vi "Test Process Register For Broadcast Throws Error if Process Uninitialized.vi"(8 "error in (no error)":errorcluster, 11 "Process Test in":refnum<class "Process Dev Test.lvclass">) -> (0 "error out":errorcluster, 3 "Process Test out":refnum<class "Process Dev Test.lvclass">)   [LabVIEW 2020, in "Process Dev Test.lvclass"]
uses:
  Process Dev Test.lvclass
  C:/Program Files (x86)/National Instruments/LabVIEW 2020/vi.lib/Astemes/LUnit/Test Case.lvclass
  source/Framework/Process/Process.lvclass
  source/Framework/Process/Process.lvclass/Process.ctl
  <vilib>/Astemes/LUnit/Test Case.lvclass/Test Case.ctl
  <vilib>/Astemes/LUnit/LUnit Assertion Result.lvclass/LUnit Assertion Result.ctl
  <vilib>/Astemes/LUnit/LUnit Test Case Result.lvclass/LUnit Test Case Result.ctl
  <vilib>/Astemes/LUnit/LUnit Method Result.lvclass/LUnit Method Result.ctl
  source/Framework/Process/Public/Lifecycle/Get Lifecycle State.vi
  <vilib>/Astemes/LUnit/Palette/Fail.vi
  <vilib>/Astemes/LUnit/Palette/Pass.vi
  <vilib>/Astemes/LUnit/Set Assertion Type.vi
  <vilib>/Utility/error.llb/Clear Errors.vi
  <vilib>/Astemes/LUnit/Add test result.vi
  <vilib>/Astemes/LUnit/LUnit Write Passed.vi
  <vilib>/Astemes/LUnit/LUnit Write Message.vi
  <vilib>/Astemes/LUnit/LUnit Write Description.vi
  <vilib>/Astemes/LUnit/LUnit Write Assertion Type.vi
  <vilib>/Astemes/LUnit/LUnit Record Assertion Result.vi
  <vilib>/Astemes/LUnit/LUnit Aggregate Assertion Results.vi
  <vilib>/Astemes/LUnit/Assertion Result/LUnit Read Status.vi
  <vilib>/Astemes/LUnit/LUnit Read Message.vi
  <vilib>/Astemes/LUnit/LUnit Read Description.vi
  <vilib>/Astemes/LUnit/Method Result/LUnit Merge Status.vi
  <vilib>/Astemes/LUnit/LUnit Concatenate result strings.vi
  <vilib>/Utility/error.llb/Error Cluster From Error Code.vi
  <vilib>/Astemes/LUnit/LUnit Assertion Result.lvclass
  <vilib>/Astemes/LUnit/Test Case.lvclass
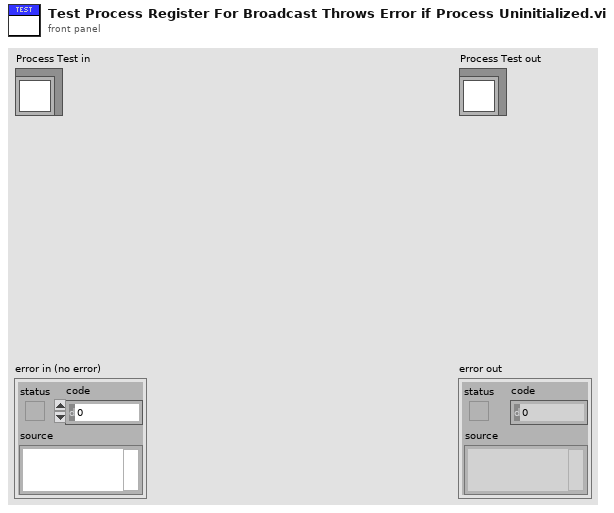
[diagram p1: front panel]
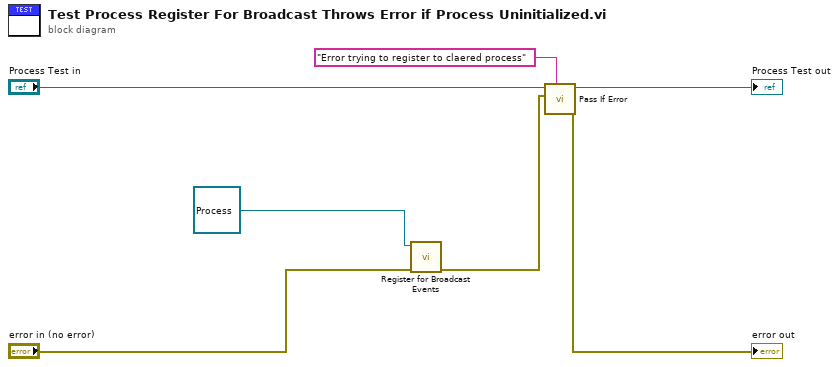
[diagram p0: block diagram]
diagram:
  n1 = call "Register for Broadcast Events.vi"("error in (no error)"="error in (no error)", "Process In"=refnum<class "Process.lvclass"> refnum ("Process.lvclass")) -> ("error out"=w2:errorcluster)  [unwired: 7 in, 2 out]
  n2 = call <vilib>:"Pass If Error.vi"("Description"="Error trying to register to claered process", "Assert error"=w2, "LUnit Test Case In"="Process Test in") -> ("error out"=→"error out":errorcluster, "LUnit Test Case Out"=→"Process Test out":refnum<class "Process Dev Test.lvclass">)  [unwired: 7 in]
